vi "BF Status.vi"() -> ()   [LabVIEW 2021]
uses:
  Controls/Bowl Feeder.ctl
panel:
  out "BF Status":T1
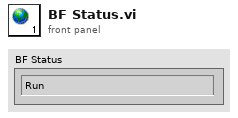
[diagram p1: front panel]
types:
  T1 = typedef "Bowl Feeder.ctl" = enum16{"Run", "Error"}
diagram:
